vi "OPC-UA_client.vi"() -> ()   [LabVIEW 2013]
uses:
  <vilib>/OPCUA/client/Read UInt32.vi
  <vilib>/OPCUA/client/Read Double.vi
  <vilib>/OPCUA/client/Write UInt32.vi
  <vilib>/OPCUA/client/Write Double.vi
  <vilib>/OPCUA/NI OPC UA Client.lvlib
panel:
  in  "update rate [ms]":dbl=100.0 format="%#_13g"
  in  "KD":dbl=0.78
  in  "KC":dbl=0.76
  in  "KB":dbl=0.76
  in  "KA":dbl=0.76
  out "VD":u32=5426850
  out "VC":u32=5580300
  out "VB":u32=5239440
  out "VA":u32=4984460
  out "MaxADC":u32=5548
  in  "Triggerlevel":u32=4000
  out "charge":dbl(graph)=88.5828
  out "charge / pC":dbl=88.5828 format="%.2f"
  out "x/mm":dbl=-0.761384 format="%.2f"
  out "y/mm":dbl=-0.237199 format="%.2f"
  out "Y-Chart":dbl(graph)=-0.237199
  out "X-Chart":dbl(graph)=-0.761384
  in  "stop":bool
  in  "node names":string[](array[string])=["Signals.SP.PosX", "Signals.SP.PosY", "Signals.SP.Charge", "DSP.DspThr1", "Signals.MaxADC", "Signals.SP.VA", "Signals.SP.VB", "Signals.SP.VC", "Signals.SP.VD", "Calibration.KA", "Calibration.KB", "Calibration.KC", "Calibration.KD"]
  in  "security policy":T1
  in  "server endpoint URL":string="opc.tcp://149.220.56.181:10021"
  # "Calibration"
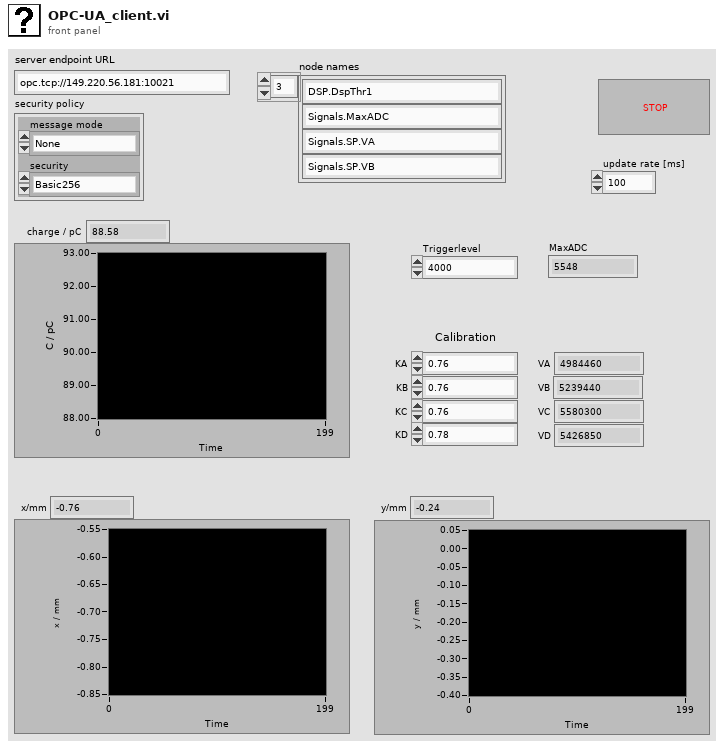
[diagram p1: front panel]
types:
  T1 = cluster{"message mode":enum16{"None", "Sign", "Sign and Encrypt"}, "security":enum16{"Basic256", "Basic128Rsa15"}}
  T2 = cluster{"Item URL":string, "Item Value":variant, "Timestamp":timestamp, "DataType":u32, "status code":u32}[]
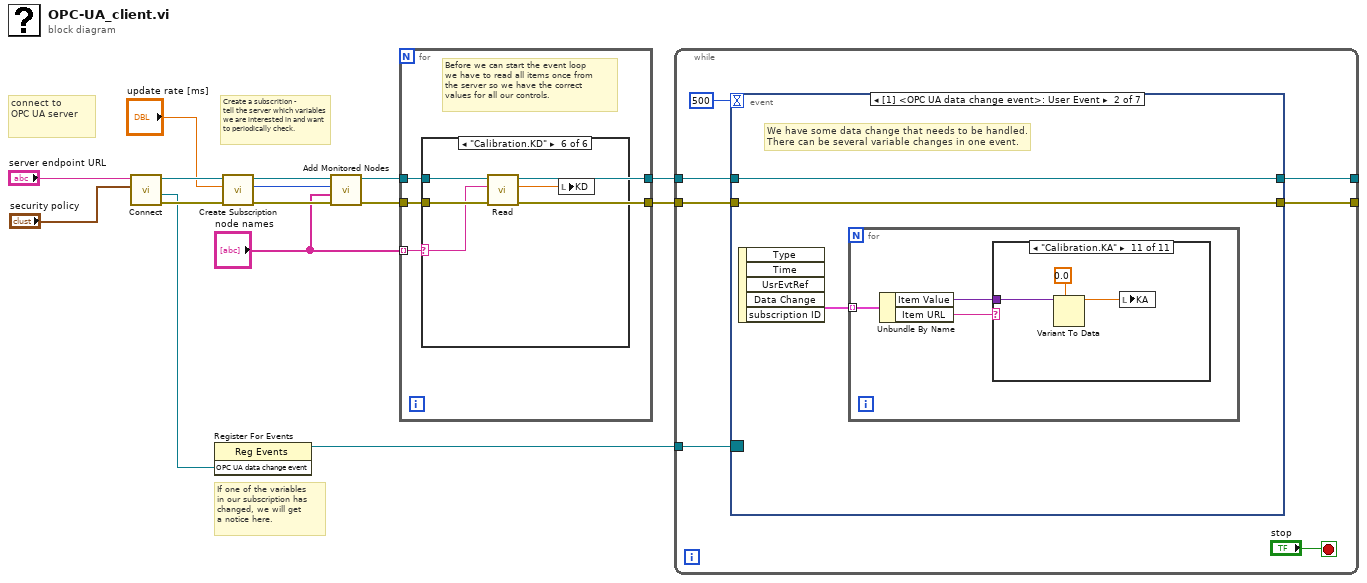
[diagram p0: block diagram]
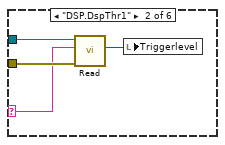
[diagram p3: hidden frame]
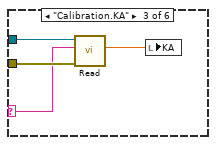
[diagram p4: hidden frame]
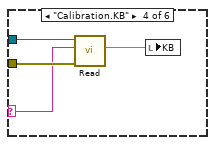
[diagram p5: hidden frame]
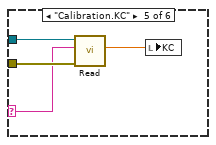
[diagram p6: hidden frame]
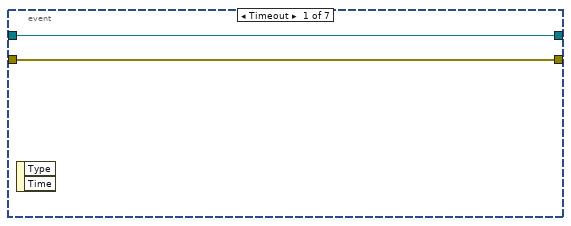
[diagram p7: hidden frame]
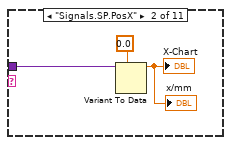
[diagram p9: hidden frame]
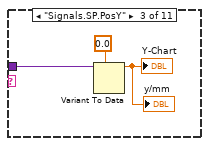
[diagram p10: hidden frame]
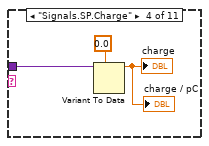
[diagram p11: hidden frame]
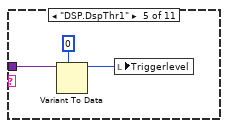
[diagram p12: hidden frame]
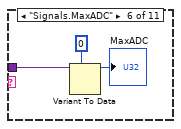
[diagram p13: hidden frame]
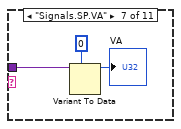
[diagram p14: hidden frame]
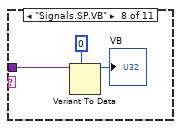
[diagram p15: hidden frame]
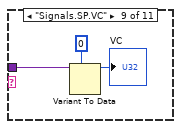
[diagram p16: hidden frame]
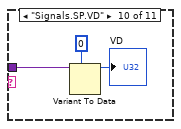
[diagram p17: hidden frame]
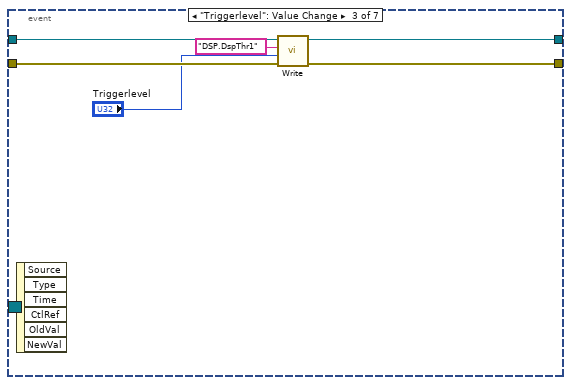
[diagram p18: hidden frame]
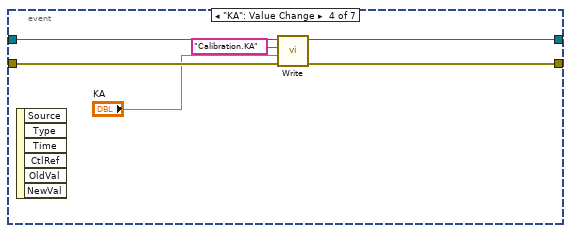
[diagram p19: hidden frame]
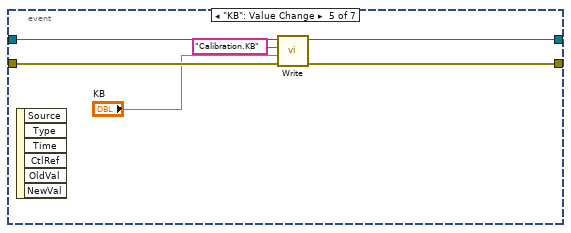
[diagram p20: hidden frame]
diagram:
  # "If one of the variables\nin our subscription has\nchanged, we will get\na notice here."
  # "Create a subscrition -\ntell the server which variables we are interested in and want to periodically check."
  # "connect to\nOPC UA server"
  n1 = call <vilib>:"Connect.vi"("security policy"="security policy", "server endpoint URL"="server endpoint URL") -> ("error out"=w12:errorcluster, "OPC UA data change event"=w7:refnum<user-event>, "OPC UA client refnum out"=w13:refnum<k21>)  [unwired: 7 in]
  n2 = register-events(w7) -> (reference out=w6:refnum<event-registration>)  [unwired: 2 in, 1 out]
  n3 = call <vilib>:"Create Subscription.vi"("error in (no error)"=w12, "update rate (1000 ms)"="update rate [ms]", "OPC UA client refnum in"=w13) -> ("error out"=w8:errorcluster, "subscription ID out"=w9:u32, "OPC UA client refnum out"=w10:refnum<k21>)  [unwired: 6 in]
  n4 = call <vilib>:"Add Monitored Nodes.vi"("error in (no error)"=w8, "array of node path"="node names", "subscription ID in"=w9, "OPC UA client refnum in"=w10) -> ("error out"=w3:errorcluster, "OPC UA client refnum out"=w4:refnum<k21>)  [unwired: 5 in, 1 out]
  n5 = for {
    tunnel: "node names" -> [w18] mode=indexing
    tunnel: w4 -> [w17]
    tunnel: w3 -> [w16]
    tunnel: [w17] -> w2
    tunnel: [w16] -> w1
    # "Before we can start the event loop\nwe have to read all items once from\nthe server so we have the correct\nvalues for all our controls."
    n6 = case shown="\"Calibration.KD\"" w18 {
      selector: w18 -> [_ w20 w24 w28 w32 w36]
      tunnel: w17 -> [_ w22 w26 w30 w34 w38]
      tunnel: w16 -> [_ w21 w25 w29 w33 w37]
      frame "False", Default {
      }
      frame "DSP.DspThr1" {
        n7 = call-poly <vilib>:"Read.vi"("error in (no error)"=w21, "node path"=w20, "OPC UA client refnum in"=w22) -> ("value"=w19:u32)  [unwired: 4 in, 4 out]
        n8 = local write "Triggerlevel"(w19) -> ()
      }
      frame "Calibration.KA" {
        n9 = call-poly <vilib>:"Read.vi"("error in (no error)"=w25, "node path"=w24, "OPC UA client refnum in"=w26) -> ("value"=w23:dbl)  [unwired: 4 in, 4 out]
        n10 = local write "KA"(w23) -> ()
      }
      frame "Calibration.KB" {
        n11 = call-poly <vilib>:"Read.vi"("error in (no error)"=w29, "node path"=w28, "OPC UA client refnum in"=w30) -> ("value"=w27:dbl)  [unwired: 4 in, 4 out]
        n12 = local write "KB"(w27) -> ()
      }
      frame "Calibration.KC" {
        n13 = call-poly <vilib>:"Read.vi"("error in (no error)"=w33, "node path"=w32, "OPC UA client refnum in"=w34) -> ("value"=w31:dbl)  [unwired: 4 in, 4 out]
        n14 = local write "KC"(w31) -> ()
      }
      frame "Calibration.KD" {
        n15 = call-poly <vilib>:"Read.vi"("error in (no error)"=w37, "node path"=w36, "OPC UA client refnum in"=w38) -> ("value"=w35:dbl)  [unwired: 4 in, 4 out]
        n16 = local write "KD"(w35) -> ()
      }
    }
  }
  n17 = while {
    tunnel: w6 -> [w45]
    tunnel: w2 -> [w43]
    tunnel: w1 -> [w42]
    tunnel: [w41] -> _
    tunnel: [w40] -> _
    stop <- "stop" stop-if-true
    n18 = event shown="[1] <OPC UA data change event>: User Event" {
      selector: w45 -> [_ _ _ _ _ _ _]
      dyn-events: _ -> [_ _ _ _ _ _ _]
      timeout: 500 -> [_ _ _ _ _ _ _]
      tunnel: w43 -> [w47 w50 w89 w95 w101 w107 w113]
      tunnel: w42 -> [w46 w49 w87 w93 w99 w105 w111]
      tunnel: [w47 w50 w88 w94 w100 w106 w112] -> w41
      tunnel: [w46 w49 w86 w92 w98 w104 w110] -> w40
      event Timeout {
        n19 = event-data() -> ()  [unwired: 1 in, 2 out]
      }
      event User Event {
        # "We have some data change that needs to be handled.\nThere can be several variable changes in one event."
        n20 = event-data() -> ("Data Change"=w48:T2)  [unwired: 1 in, 4 out]
        n21 = for {
          tunnel: w48 -> [w53] mode=indexing
          n22 = Unbundle By Name(w53) -> ("Item Value"=w51:variant, "Item URL"=w52:string)
          n23 = case shown="\"Calibration.KA\"" w52 {
            tunnel: w51 -> [_ w54 w57 w60 w64 w67 w70 w73 w76 w79 w82]
            frame "False", Default {
            }
            frame "Signals.SP.PosX" {
              n24 = Variant To Data(type=0.0, Variant=w54) -> (data=→"X-Chart" →"x/mm":dbl)  [unwired: 1 in, 1 out]
            }
            frame "Signals.SP.PosY" {
              n25 = Variant To Data(type=0.0, Variant=w57) -> (data=→"Y-Chart" →"y/mm":dbl)  [unwired: 1 in, 1 out]
            }
            frame "Signals.SP.Charge" {
              n26 = Variant To Data(type=0.0, Variant=w60) -> (data=→"charge" →"charge / pC":dbl)  [unwired: 1 in, 1 out]
            }
            frame "DSP.DspThr1" {
              n27 = Variant To Data(type=u32 0, Variant=w64) -> (data=w63:u32)  [unwired: 1 in, 1 out]
              n28 = local write "Triggerlevel"(w63) -> ()
            }
            frame "Signals.MaxADC" {
              n29 = Variant To Data(type=u32 0, Variant=w67) -> (data=→"MaxADC":u32)  [unwired: 1 in, 1 out]
            }
            frame "Signals.SP.VA" {
              n30 = Variant To Data(type=u32 0, Variant=w70) -> (data=→"VA":u32)  [unwired: 1 in, 1 out]
            }
            frame "Signals.SP.VB" {
              n31 = Variant To Data(type=u32 0, Variant=w73) -> (data=→"VB":u32)  [unwired: 1 in, 1 out]
            }
            frame "Signals.SP.VC" {
              n32 = Variant To Data(type=u32 0, Variant=w76) -> (data=→"VC":u32)  [unwired: 1 in, 1 out]
            }
            frame "Signals.SP.VD" {
              n33 = Variant To Data(type=u32 0, Variant=w79) -> (data=→"VD":u32)  [unwired: 1 in, 1 out]
            }
            frame "Calibration.KA" {
              n34 = Variant To Data(type=0.0, Variant=w82) -> (data=w81:dbl)  [unwired: 1 in, 1 out]
              n35 = local write "KA"(w81) -> ()
            }
          }
        }
      }
      event "Triggerlevel": Value Change {
        n36 = event-data() -> ()  [unwired: 1 in, 6 out]
        n37 = call-poly <vilib>:"Write.vi"("error in (no error)"=w87, "value"="Triggerlevel", "node path"="DSP.DspThr1", "OPC UA client refnum in"=w89) -> ("error out"=w86:errorcluster, "OPC UA client refnum out"=w88:refnum<k21>)  [unwired: 5 in, 1 out]
      }
      event "KA": Value Change {
        n38 = event-data() -> ()  [unwired: 1 in, 6 out]
        n39 = call-poly <vilib>:"Write.vi"("error in (no error)"=w93, "value"="KA", "node path"="Calibration.KA", "OPC UA client refnum in"=w95) -> ("error out"=w92:errorcluster, "OPC UA client refnum out"=w94:refnum<k21>)  [unwired: 5 in, 1 out]
      }
      event "KB": Value Change {
        n40 = event-data() -> ()  [unwired: 1 in, 6 out]
        n41 = call-poly <vilib>:"Write.vi"("error in (no error)"=w99, "value"="KB", "node path"="Calibration.KB", "OPC UA client refnum in"=w101) -> ("error out"=w98:errorcluster, "OPC UA client refnum out"=w100:refnum<k21>)  [unwired: 5 in, 1 out]
      }
      event "KC": Value Change {
        n42 = event-data() -> ()  [unwired: 1 in, 6 out]
        n43 = call-poly <vilib>:"Write.vi"("error in (no error)"=w105, "value"="KC", "node path"="Calibration.KC", "OPC UA client refnum in"=w107) -> ("error out"=w104:errorcluster, "OPC UA client refnum out"=w106:refnum<k21>)  [unwired: 5 in, 1 out]
      }
      event "KD": Value Change {
        n44 = event-data() -> ()  [unwired: 1 in, 6 out]
        n45 = call-poly <vilib>:"Write.vi"("error in (no error)"=w111, "value"="KD", "node path"="Calibration.KD", "OPC UA client refnum in"=w113) -> ("error out"=w110:errorcluster, "OPC UA client refnum out"=w112:refnum<k21>)  [unwired: 5 in, 1 out]
      }
    }
  }
